vi "Get image date.vi"(8 "error in (no error)":errorcluster, 11 "Simulated_CCD_Camera in":refnum<class "Sim_Ixon_Ultra.lvclass">) -> (0 "error out":errorcluster, 3 "Simulated_CCD_Camera out":refnum<class "Sim_Ixon_Ultra.lvclass">)   [LabVIEW 2018, in "Sim_Ixon_Ultra.lvclass"]
doc: "Get the time stamp (in UTC) at star of exposure"
uses:
  Sim_Ixon_Ultra.lvclass
  Sim_Ixon_Ultra.lvclass/Sim_Ixon_Ultra.ctl
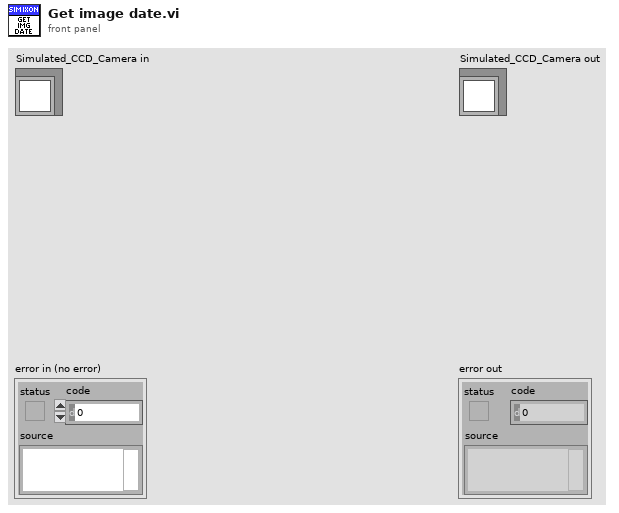
[diagram p1: front panel]
types:
  T1 = typedef "LVDateTimeRec.ctl" = cluster{"fractional second":dbl, "second":i32, "minute":i32, "hour":i32, "day of month":i32, "month":i32, "year":i32, "day of week":i32, "day of year":i32, "DST":i32}
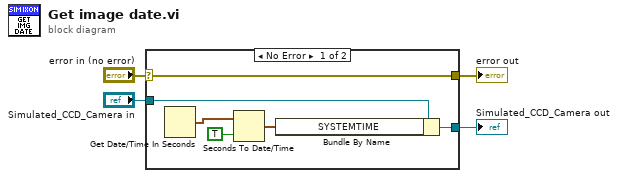
[diagram p0: block diagram]
diagram:
  n1 = case shown="No Error" "error in (no error)" {
    selector: "error in (no error)" -> [w10 w12]
    tunnel: [w10 w12] -> w3
    tunnel: [w7 w11] -> w1
    tunnel: "Simulated_CCD_Camera in" -> [w8 w11]
    frame No Error {
      n2 = Get Date/Time In Seconds() -> (seconds since 1Jan1904=w9:timestamp)
      n3 = Seconds To Date/Time(time stamp (now)=w9, to UTC (F)=TRUE) -> (date time rec=w5:T1)
      n4 = Bundle By Name(cluster=w8, "SYSTEMTIME"=w5) -> (w7:refnum<class "Sim_Ixon_Ultra.lvclass">)
    }
    frame Error {
    }
  }
  "error out" <- w3
  "Simulated_CCD_Camera out" <- w1
